vi "Initialize.vi"   [LabVIEW 2011]
uses:
  Controls/Device Cluster.ctl
  GlobalVariables.vi
types:
  T1 = typedef "GP275 Cluster.ctl" = cluster{"Pressure (Torr)":sgl}
  T2 = typedef "RTPC Cluster.ctl" = cluster{"ID Number":u8, "Status":bool[], "Flow (SCCM)":dbl, "Pressure (SCCM)":dbl, "Valve":i16, "Active Instance":i8, "Output":dbl}
  T3 = typedef "MFC Cluster.ctl" = cluster{"ID Number":u8, "Status":bool[], "Flow (SCCM)":dbl, "SetPoint (SCCM)":dbl, "Actuator Override":i8, "Actuator Drive Valve":i16, "Setpoint Output":dbl}
  T4 = typedef "BAR Cluster.ctl" = cluster{"Pressure":dbl}
  T5 = typedef "PC Cluster.ctl" = cluster{"ID Number":u8, "Status":bool[], "Flow (SCCM)":dbl, "SetPoint (SCCM)":dbl, "Actuator Override":i8, "Actuator Drive Valve":i16, "Setpoint Output":dbl}
  T6 = typedef "Device Cluster.ctl" = cluster{"Dnet":string, "Node":i32, "Type":string, "ID Number":u8, "SCCM":dbl, "FullScale":dbl, "Input Bytes":i32, "Output Bytes":i32, "Input Start Location":i32, "Output Start Location":i32, "Enabled":bool, "Bytes":u8[]}
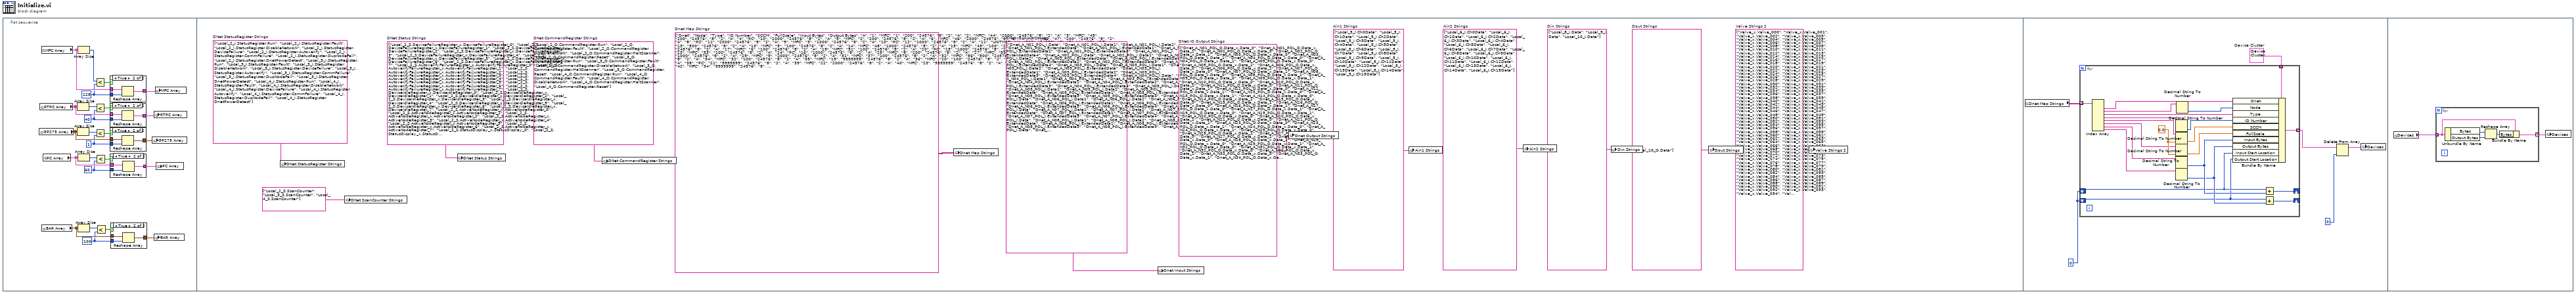
[diagram p0: block diagram]
diagram:
  n1 = flat-sequence {
    frame #0 {
      w2 = 60 ("y")
      w10 = 100 ("y")
      w14 = 1 ("y")
      w18 = 40 ("y")
      w22 = 128 ("y")
      n2 = global read "GlobalVariables.vi" "GP275 Array"() -> (w15:T1[])
      n3 = global read "GlobalVariables.vi" "RTPC Array"() -> (w19:T2[])
      n4 = global read "GlobalVariables.vi" "MFC Array"() -> (w23:T3[])
      n5 = global read "GlobalVariables.vi" "BAR Array"() -> (w11:T4[])
      n6 = global read "GlobalVariables.vi" "PC Array"() -> (w3:T5[])
      n7 = Array Size(array=w19) -> (size(s)=w21:i32)
      n8 = Array Size(array=w15) -> (size(s)=w17:i32)
      n9 = Array Size(array=w3) -> (size(s)=w5:i32)
      n10 = Array Size(array=w23) -> (size(s)=w25:i32)
      n11 = Array Size(array=w11) -> (size(s)=w13:i32)
      n12 = Less?(x=w25, y=w22) -> (x < y?=w24:bool)
      n13 = Less?(x=w21, y=w18) -> (x < y?=w20:bool)
      n14 = Less?(x=w17, y=w14) -> (x < y?=w16:bool)
      n15 = Less?(x=w5, y=w2) -> (x < y?=w4:bool)
      n16 = Less?(x=w13, y=w10) -> (x < y?=w12:bool)
      n17 = case shown="True" w24 {
        tunnel: w23 -> [w42 w45]
        tunnel: w22 -> [_ w44]
        tunnel: [w42 w43] -> w9
        frame False {
        }
        frame True {
          n18 = Reshape Array(w45, w44) -> (w43:T3[])
        }
      }
      n19 = case shown="True" w20 {
        tunnel: w19 -> [w38 w41]
        tunnel: w18 -> [_ w40]
        tunnel: [w38 w39] -> w8
        frame False {
        }
        frame True {
          n20 = Reshape Array(w41, w40) -> (w39:T2[])
        }
      }
      n21 = case shown="True" w16 {
        tunnel: w15 -> [w34 w37]
        tunnel: w14 -> [_ w36]
        tunnel: [w34 w35] -> w7
        frame False {
        }
        frame True {
          n22 = Reshape Array(w37, w36) -> (w35:T1[])
        }
      }
      n23 = case shown="True" w4 {
        tunnel: w3 -> [w26 w29]
        tunnel: w2 -> [_ w28]
        tunnel: [w26 w27] -> w1
        frame False {
        }
        frame True {
          n24 = Reshape Array(w29, w28) -> (w27:T5[])
        }
      }
      n25 = case shown="True" w12 {
        tunnel: w11 -> [w30 w33]
        tunnel: w10 -> [_ w32]
        tunnel: [w30 w31] -> w6
        frame False {
        }
        frame True {
          n26 = Reshape Array(w33, w32) -> (w31:T4[])
        }
      }
      n27 = global write "GlobalVariables.vi" "GP275 Array"(w7) -> ()
      n28 = global write "GlobalVariables.vi" "RTPC Array"(w8) -> ()
      n29 = global write "GlobalVariables.vi" "BAR Array"(w6) -> ()
      n30 = global write "GlobalVariables.vi" "MFC Array"(w9) -> ()
      n31 = global write "GlobalVariables.vi" "PC Array"(w1) -> ()
    }
    frame #1 {
      w47 = string[] ["Dnet_A_N01_POL_O.Data_x.Data_0", "Dnet_A_N01_POL_O.Data_x.Data_1", "Dnet_A_N02_POL_O.Data_x.Data_0", "Dnet_A_N02_POL_O.Data_x.Data_1", "Dnet_A_N03_POL_O.Data_x.Data_0", "Dnet_A_N03_POL_O.Data_x.Data_1", "Dnet_A_N04_POL_O.Data_x.Data_0", "Dnet_A_N04_POL_O.Data_x.Data_1", "Dnet_A_N05_POL_O.Data_x.Data_0", "Dnet_A_N05_POL_O.Data_x.Data_1", "Dnet_A_N06_POL_O.Data_x.Data_0", "Dnet_A_N06_POL_O.Data_x.Data_1", "Dnet_A_N07_POL_O.Data_x.Data_0", "Dnet_A_N07_POL_O.Data_x.Data_1", "Dnet_A_N08_POL_O.Data_x.Data_0", "Dnet_A_N08_POL_O.Data_x.Data_1", "Dnet_A_N09_POL_O.Data_x.Data_0", "Dnet_A_N09_POL_O.Data_x.Data_1", "Dnet_A_N10_POL_O.Data_x.Data_0", "Dnet_A_N10_POL_O.Data_x.Data_1", "Dnet_A_N11_POL_O.Data_x.Data_0", "Dnet_A_N11_POL_O.Data_x.Data_1", "Dnet_A_N12_POL_O.Data_x.Data_0", "Dnet_A_N12_POL_O.Data_x.Data_1", "Dnet_A_N13_POL_O.Data_x.Data_0", "Dnet_A_N13_POL_O.Data_x.Data_1", "Dnet_A_N14_POL_O.Data_x.Data_0", "Dnet_A_N14_POL_O.Data_x.Data_1", "Dnet_A_N15_POL_O.Data_x.Data_0", "Dnet_A_N15_POL_O.Data_x.Data_1", "Dnet_A_N16_POL_O.Data_x.Data_0", "Dnet_A_N16_POL_O.Data_x.Data_1", "Dnet_A_N17_POL_O.Data_x.Data_0", "Dnet_A_N17_POL_O.Data_x.Data_1", "Dnet_A_N19_POL_O.Data_x.Data_0", "Dnet_A_N19_POL_O.Data_x.Data_1", "Dnet_A_N20_POL_O.Data_x.Data_0", "Dnet_A_N20_POL_O.Data_x.Data_1", "Dnet_A_N21_POL_O.Data_x.Data_0", "Dnet_A_N21_POL_O.Data_x.Data_1", "Dnet_A_N23_POL_O.Data_x.Data_0", "Dnet_A_N23_POL_O.Data_x.Data_1", "Dnet_A_N24_POL_O.Data_x.Data_0", "Dnet_A_N24_POL_O.Data_x.Data_1", "Dnet_A_N25_POL_O.Data_x.Data_0", "Dnet_A_N25_POL_O.Data_x.Data_1", "Dnet_A_N27_POL_O.Data_x.Data_0", "Dnet_A_N27_POL_O.Data_x.Data_1", "Dnet_A_N28_POL_O.Data_x.Data_0", "Dnet_A_N28_POL_O.Data_x.Data_1", "Dnet_A_N29_POL_O.Data_x.Data_0", "Dnet_A_N29_POL_O.Data_x.Data_1", "Dnet_A_N31_POL_O.Data_x.Data_0", "Dnet_A_N31_POL_O.Data_x.Data_1", "Dnet_A_N32_POL_O.Data_x.Data_0", "Dnet_A_N32_POL_O.Data_x.Data_1", "Dnet_A_N33_POL_O.Data_x.Data_0", "Dnet_A_N33_POL_O.Data_x.Data_1", "Dnet_A_N34_POL_O.Data_x.Data_0", "Dnet_A_N34_POL_O.Data_x.Data_1", "Dnet_A_N35_POL_O.Data_x.Data_0", "Dnet_A_N35_POL_O.Data_x.Data_1", "Dnet_A_N36_POL_O.Data_x.Data_0", "Dnet_A_N36_POL_O.Data_x.Data_1", "Dnet_A_N37_POL_O.Data_x.Data_0", "Dnet_A_N37_POL_O.Data_x.Data_1", "Dnet_A_N38_POL_O.Data_x.Data_0", "Dnet_A_N38_POL_O.Data_x.Data_1", "Dnet_A_N39_POL_O.Data_x.Data_0", "Dnet_A_N39_POL_O.Data_x.Data_1", "Dnet_A_N40_POL_O.Data_x.Data_0", "Dnet_A_N40_POL_O.Data_x.Data_1", "Dnet_A_N41_POL_O.Data_x.Data_0", "Dnet_A_N41_POL_O.Data_x.Data_1", "Dnet_A_N42_POL_O.Data_x.Data_0", "Dnet_A_N42_POL_O.Data_x.Data_1", "Dnet_A_N43_POL_O.Data_x.Data_0", "Dnet_A_N43_POL_O.Data_x.Data_1", "Dnet_A_N44_POL_O.Data_x.Data_0", "Dnet_A_N44_POL_O.Data_x.Data_1", "Dnet_A_N45_POL_O.Data_x.Data_0", "Dnet_A_N45_POL_O.Data_x.Data_1", "Dnet_A_N46_POL_O.Data_x.Data_0", "Dnet_A_N46_POL_O.Data_x.Data_1", "Dnet_A_N47_POL_O.Data_x.Data_0", "Dnet_A_N47_POL_O.Data_x.Data_1", "Dnet_A_N49_POL_O.Data", "Dnet_A_N49_POL_O.Data1", "Dnet_A_N49_POL_O.ExtendedData", "Dnet_A_N50_POL_O.Data_x.Data_0", "Dnet_A_N50_POL_O.Data_x.Data_1", "Dnet_A_N51_POL_O.Data_x.Data_0", "Dnet_A_N51_POL_O.Data_x.Data_1", "Dnet_A_N52_POL_O.Data", "Dnet_A_N52_POL_O.Data1", "Dnet_A_N52_POL_O.ExtendedData", "Dnet_A_N53_POL_O.Data", "Dnet_A_N53_POL_O.Data1", "Dnet_A_N53_POL_O.ExtendedData", "Dnet_A_N54_POL_O.Data", "Dnet_A_N54_POL_O.Data1", "Dnet_A_N54_POL_O.ExtendedData", "Dnet_A_N55_POL_O.Data_x.Data_0", "Dnet_A_N55_POL_O.Data_x.Data_1", "Dnet_A_N56_POL_O.Data_x.Data_0", "Dnet_A_N56_POL_O.Data_x.Data_1", "Dnet_A_N60_POL_O.Data_x.Data_0", "Dnet_A_N60_POL_O.Data_x.Data_1", "Dnet_A_N60_POL_O.Data_x.Data_2", "Dnet_A_N60_POL_O.Data_x.Data_3", "Dnet_A_N60_POL_O.Data_x.Data_4", "Dnet_A_N60_POL_O.Data_x.Data_5", "Dnet_A_N60_POL_O.Data_x.Data_6", "Dnet_A_N60_POL_O.Data_x.Data_7", "Dnet_A_N63_POL_O.Data_x.Data_0", "Dnet_A_N63_POL_O.Data_x.Data_1", "Dnet_B_N01_POL_O.Data_x.Data_0", "Dnet_B_N01_POL_O.Data_x.Data_1", "Dnet_B_N02_POL_O.Data_x.Data_0", "Dnet_B_N02_POL_O.Data_x.Data_1", "Dnet_B_N03_POL_O.Data_x.Data_0", "Dnet_B_N03_POL_O.Data_x.Data_1", "Dnet_B_N04_POL_O.Data_x.Data_0", "Dnet_B_N04_POL_O.Data_x.Data_1", "Dnet_B_N05_POL_O.Data_x.Data_0", "Dnet_B_N05_POL_O.Data_x.Data_1", "Dnet_B_N06_POL_O.Data_x.Data_0", "Dnet_B_N06_POL_O.Data_x.Data_1", "Dnet_B_N08_POL_O.Data_x.Data_0", "Dnet_B_N08_POL_O.Data_x.Data_1", "Dnet_B_N09_POL_O.Data_x.Data_0", "Dnet_B_N09_POL_O.Data_x.Data_1", "Dnet_B_N10_POL_O.Data_x.Data_0", "Dnet_B_N10_POL_O.Data_x.Data_1", "Dnet_B_N11_POL_O.Data_x.Data_0", "Dnet_B_N11_POL_O.Data_x.Data_1", "Dnet_B_N12_POL_O.Data_x.Data_0", "Dnet_B_N12_POL_O.Data_x.Data_1", "Dnet_B_N13_POL_O.Data_x.Data_0", "Dnet_B_N13_POL_O.Data_x.Data_1", "Dnet_B_N14_POL_O.Data_x.Data_0", "Dnet_B_N14_POL_O.Data_x.Data_1", "Dnet_B_N15_POL_O.Data_x.Data_0", "Dnet_B_N15_POL_O.Data_x.Data_1", "Dnet_B_N21_POL_O.Data", "Dnet_C_N09_POL_O.Data_x.Data_00", "Dnet_C_N09_POL_O.Data_x.Data_01", "Dnet_C_N09_POL_O.Data_x.Data_02", "Dnet_C_N09_POL_O.Data_x.Data_03", "Dnet_C_N09_POL_O.Data_x.Data_04", "Dnet_C_N09_POL_O.Data_x.Data_05", "Dnet_C_N09_POL_O.Data_x.Data_06", "Dnet_C_N09_POL_O.Data_x.Data_07", "Dnet_C_N09_POL_O.Data_x.Data_08", "Dnet_C_N09_POL_O.Data_x.Data_09", "Dnet_C_N09_POL_O.Data_x.Data_10", "Dnet_C_N09_POL_O.Data_x.Data_11", "Dnet_C_N09_POL_O.Data_x.Data_12", "Dnet_C_N09_POL_O.Data_x.Data_13", "Dnet_C_N09_POL_O.Data_x.Data_14", "Dnet_C_N09_POL_O.Data_x.Data_15", "Dnet_C_N09_POL_O.Data_x.Data_16", "Dnet_C_N09_POL_O.Data_x.Data_17", "Dnet_C_N09_POL_O.Data_x.Data_18", "Dnet_C_N09_POL_O.Data_x.Data_19", "Dnet_C_N09_POL_O.Data_x.Data_20", "Dnet_C_N09_POL_O.Data_x.Data_21", "Dnet_C_N09_POL_O.Data_x.Data_22", "Dnet_C_N09_POL_O.Data_x.Data_23", "Dnet_C_N09_POL_O.Data_x.Data_24", "Dnet_C_N09_POL_O.Data_x.Data_25", "Dnet_C_N09_POL_O.Data_x.Data_26", "Dnet_C_N09_POL_O.Data_x.Data_27", "Dnet_C_N09_POL_O.Data_x.Data_28", "Dnet_C_N09_POL_O.Data_x.Data_29", "Dnet_C_N09_POL_O.Data_x.Data_30", "Dnet_C_N09_POL_O.Data_x.Data_31", "Dnet_C_N09_POL_O.Data_x.Data_32", "Dnet_C_N09_POL_O.Data_x.Data_33", "Dnet_C_N09_POL_O.Data_x.Data_34", "Dnet_C_N09_POL_O.Data_x.Data_35", "Dnet_C_N09_POL_O.Data_x.Data_36", "Dnet_C_N09_POL_O.Data_x.Data_37", "Dnet_C_N09_POL_O.Data_x.Data_38", "Dnet_C_N09_POL_O.Data_x.Data_39", "Dnet_C_N09_POL_O.Data_x.Data_40", "Dnet_C_N09_POL_O.Data_x.Data_41", "Dnet_C_N09_POL_O.Data_x.Data_42", "Dnet_C_N09_POL_O.Data_x.Data_43", "Dnet_C_N09_POL_O.Data_x.Data_44", "Dnet_C_N09_POL_O.Data_x.Data_45", "Dnet_C_N09_POL_O.Data_x.Data_46", "Dnet_C_N09_POL_O.Data_x.Data_47", "Dnet_C_N09_POL_O.Data_x.Data_48", "Dnet_C_N09_POL_O.Data_x.Data_49", "Dnet_C_N09_POL_O.Data_x.Data_50", "Dnet_C_N09_POL_O.Data_x.Data_51", "Dnet_C_N09_POL_O.Data_x.Data_52", "Dnet_C_N09_POL_O.Data_x.Data_53", "Dnet_C_N09_POL_O.Data_x.Data_54", "Dnet_C_N09_POL_O.Data_x.Data_55", "Dnet_C_N09_POL_O.Data_x.Data_56", "Dnet_C_N09_POL_O.Data_x.Data_57", "Dnet_C_N09_POL_O.Data_x.Data_58", "Dnet_C_N09_POL_O.Data_x.Data_59", "Dnet_C_N09_POL_O.Data_x.Data_60", "Dnet_C_N09_POL_O.Data_x.Data_61", "Dnet_C_N09_POL_O.Data_x.Data_62", "Dnet_C_N09_POL_O.Data_x.Data_63", "Dnet_C_N09_POL_O.Data_x.Data_64", "Dnet_C_N09_POL_O.Data_x.Data_65", "Dnet_C_N09_POL_O.Data_x.Data_66", "Dnet_C_N09_POL_O.Data_x.Data_67", "Dnet_C_N09_POL_O.Data_x.Data_68", "Dnet_C_N09_POL_O.Data_x.Data_69", "Dnet_C_N09_POL_O.Data_x.Data_70", "Dnet_C_N09_POL_O.Data_x.Data_71", "Dnet_C_N09_POL_O.Data_x.Data_72", "Dnet_C_N09_POL_O.Data_x.Data_73", "Dnet_C_N09_POL_O.Data_x.Data_74", "Dnet_C_N09_POL_O.Data_x.Data_75", "Dnet_C_N09_POL_O.Data_x.Data_76", "Dnet_C_N09_POL_O.Data_x.Data_77", "Dnet_C_N09_POL_O.Data_x.Data_78", "Dnet_C_N09_POL_O.Data_x.Data_79"]  # DNet IO Output Strings
      w46 = string[] ["Dnet_A_N01_POL_I.Data", "Dnet_A_N01_POL_I.Data1", "Dnet_A_N01_POL_I.Data2", "Dnet_A_N01_POL_I.ExtendedData", "Dnet_A_N01_POL_I.ExtendedData1", "Dnet_A_N01_POL_I.ExtendedData2", "Dnet_A_N01_POL_I.ExtendedData3", "Dnet_A_N01_POL_I.ExtendedData4", "Dnet_A_N02_POL_I.Data", "Dnet_A_N02_POL_I.Data1", "Dnet_A_N02_POL_I.Data2", "Dnet_A_N02_POL_I.ExtendedData", "Dnet_A_N02_POL_I.ExtendedData1", "Dnet_A_N02_POL_I.ExtendedData2", "Dnet_A_N02_POL_I.ExtendedData3", "Dnet_A_N02_POL_I.ExtendedData4", "Dnet_A_N03_POL_I.Data", "Dnet_A_N03_POL_I.Data1", "Dnet_A_N03_POL_I.Data2", "Dnet_A_N03_POL_I.ExtendedData", "Dnet_A_N03_POL_I.ExtendedData1", "Dnet_A_N03_POL_I.ExtendedData2", "Dnet_A_N03_POL_I.ExtendedData3", "Dnet_A_N03_POL_I.ExtendedData4", "Dnet_A_N04_POL_I.Data", "Dnet_A_N04_POL_I.Data1", "Dnet_A_N04_POL_I.Data2", "Dnet_A_N04_POL_I.ExtendedData", "Dnet_A_N04_POL_I.ExtendedData1", "Dnet_A_N04_POL_I.ExtendedData2", "Dnet_A_N04_POL_I.ExtendedData3", "Dnet_A_N04_POL_I.ExtendedData4", "Dnet_A_N05_POL_I.Data", "Dnet_A_N05_POL_I.Data1", "Dnet_A_N05_POL_I.Data2", "Dnet_A_N05_POL_I.ExtendedData", "Dnet_A_N05_POL_I.ExtendedData1", "Dnet_A_N05_POL_I.ExtendedData2", "Dnet_A_N05_POL_I.ExtendedData3", "Dnet_A_N05_POL_I.ExtendedData4", "Dnet_A_N06_POL_I.Data", "Dnet_A_N06_POL_I.Data1", "Dnet_A_N06_POL_I.Data2", "Dnet_A_N06_POL_I.ExtendedData", "Dnet_A_N06_POL_I.ExtendedData1", "Dnet_A_N06_POL_I.ExtendedData2", "Dnet_A_N06_POL_I.ExtendedData3", "Dnet_A_N06_POL_I.ExtendedData4", "Dnet_A_N07_POL_I.Data", "Dnet_A_N07_POL_I.Data1", "Dnet_A_N07_POL_I.Data2", "Dnet_A_N07_POL_I.ExtendedData", "Dnet_A_N07_POL_I.ExtendedData1", "Dnet_A_N07_POL_I.ExtendedData2", "Dnet_A_N07_POL_I.ExtendedData3", "Dnet_A_N07_POL_I.ExtendedData4", "Dnet_A_N08_POL_I.Data", "Dnet_A_N08_POL_I.Data1", "Dnet_A_N08_POL_I.Data2", "Dnet_A_N08_POL_I.ExtendedData", "Dnet_A_N08_POL_I.ExtendedData1", "Dnet_A_N08_POL_I.ExtendedData2", "Dnet_A_N08_POL_I.ExtendedData3", "Dnet_A_N08_POL_I.ExtendedData4", "Dnet_A_N09_POL_I.Data", "Dnet_A_N09_POL_I.Data1", "Dnet_A_N09_POL_I.Data2", "Dnet_A_N09_POL_I.ExtendedData", "Dnet_A_N09_POL_I.ExtendedData1", "Dnet_A_N09_POL_I.ExtendedData2", "Dnet_A_N09_POL_I.ExtendedData3", "Dnet_A_N09_POL_I.ExtendedData4", "Dnet_A_N10_POL_I.Data", "Dnet_A_N10_POL_I.Data1", "Dnet_A_N10_POL_I.Data2", "Dnet_A_N10_POL_I.ExtendedData", "Dnet_A_N10_POL_I.ExtendedData1", "Dnet_A_N10_POL_I.ExtendedData2", "Dnet_A_N10_POL_I.ExtendedData3", "Dnet_A_N10_POL_I.ExtendedData4", "Dnet_A_N11_POL_I.Data_x.Data_0", "Dnet_A_N11_POL_I.Data_x.Data_1", "Dnet_A_N11_POL_I.Data_x.Data_2", "Dnet_A_N11_POL_I.Data_x.Data_3", "Dnet_A_N11_POL_I.Data_x.Data_4", "Dnet_A_N11_POL_I.Data_x.Data_5", "Dnet_A_N11_POL_I.Data_x.Data_6", "Dnet_A_N11_POL_I.Data_x.Data_7", "Dnet_A_N12_POL_I.Data", "Dnet_A_N12_POL_I.Data1", "Dnet_A_N12_POL_I.Data2", "Dnet_A_N12_POL_I.ExtendedData", "Dnet_A_N12_POL_I.ExtendedData1", "Dnet_A_N12_POL_I.ExtendedData2", "Dnet_A_N12_POL_I.ExtendedData3", "Dnet_A_N12_POL_I.ExtendedData4", "Dnet_A_N13_POL_I.Data", "Dnet_A_N13_POL_I.Data1", "Dnet_A_N13_POL_I.Data2", "Dnet_A_N13_POL_I.ExtendedData", "Dnet_A_N13_POL_I.ExtendedData1", "Dnet_A_N13_POL_I.ExtendedData2", "Dnet_A_N13_POL_I.ExtendedData3", "Dnet_A_N13_POL_I.ExtendedData4", "Dnet_A_N14_POL_I.Data", "Dnet_A_N14_POL_I.Data1", "Dnet_A_N14_POL_I.Data2", "Dnet_A_N14_POL_I.ExtendedData", "Dnet_A_N14_POL_I.ExtendedData1", "Dnet_A_N14_POL_I.ExtendedData2", "Dnet_A_N14_POL_I.ExtendedData3", "Dnet_A_N14_POL_I.ExtendedData4", "Dnet_A_N15_POL_I.Data", "Dnet_A_N15_POL_I.Data1", "Dnet_A_N15_POL_I.Data2", "Dnet_A_N15_POL_I.ExtendedData", "Dnet_A_N15_POL_I.ExtendedData1", "Dnet_A_N15_POL_I.ExtendedData2", "Dnet_A_N15_POL_I.ExtendedData3", "Dnet_A_N15_POL_I.ExtendedData4", "Dnet_A_N16_POL_I.Data", "Dnet_A_N16_POL_I.Data1", "Dnet_A_N16_POL_I.Data2", "Dnet_A_N16_POL_I.ExtendedData", "Dnet_A_N16_POL_I.ExtendedData1", "Dnet_A_N16_POL_I.ExtendedData2", "Dnet_A_N16_POL_I.ExtendedData3", "Dnet_A_N16_POL_I.ExtendedData4", "Dnet_A_N17_POL_I.Data", "Dnet_A_N17_POL_I.Data1", "Dnet_A_N17_POL_I.Data2", "Dnet_A_N17_POL_I.ExtendedData", "Dnet_A_N17_POL_I.ExtendedData1", "Dnet_A_N17_POL_I.ExtendedData2", "Dnet_A_N17_POL_I.ExtendedData3", "Dnet_A_N17_POL_I.ExtendedData4", "Dnet_A_N19_POL_I.Data", "Dnet_A_N19_POL_I.Data1", "Dnet_A_N19_POL_I.Data2", "Dnet_A_N19_POL_I.ExtendedData", "Dnet_A_N19_POL_I.ExtendedData1", "Dnet_A_N19_POL_I.ExtendedData2", "Dnet_A_N19_POL_I.ExtendedData3", "Dnet_A_N19_POL_I.ExtendedData4", "Dnet_A_N20_POL_I.Data", "Dnet_A_N20_POL_I.Data1", "Dnet_A_N20_POL_I.Data2", "Dnet_A_N20_POL_I.ExtendedData", "Dnet_A_N20_POL_I.ExtendedData1", "Dnet_A_N20_POL_I.ExtendedData2", "Dnet_A_N20_POL_I.ExtendedData3", "Dnet_A_N20_POL_I.ExtendedData4", "Dnet_A_N21_POL_I.Data", "Dnet_A_N21_POL_I.Data1", "Dnet_A_N21_POL_I.Data2", "Dnet_A_N21_POL_I.ExtendedData", "Dnet_A_N21_POL_I.ExtendedData1", "Dnet_A_N21_POL_I.ExtendedData2", "Dnet_A_N21_POL_I.ExtendedData3", "Dnet_A_N21_POL_I.ExtendedData4", "Dnet_A_N23_POL_I.Data", "Dnet_A_N23_POL_I.Data1", "Dnet_A_N23_POL_I.Data2", "Dnet_A_N23_POL_I.ExtendedData", "Dnet_A_N23_POL_I.ExtendedData1", "Dnet_A_N23_POL_I.ExtendedData2", "Dnet_A_N23_POL_I.ExtendedData3", "Dnet_A_N23_POL_I.ExtendedData4", "Dnet_A_N24_POL_I.Data", "Dnet_A_N24_POL_I.Data1", "Dnet_A_N24_POL_I.Data2", "Dnet_A_N24_POL_I.ExtendedData", "Dnet_A_N24_POL_I.ExtendedData1", "Dnet_A_N24_POL_I.ExtendedData2", "Dnet_A_N24_POL_I.ExtendedData3", "Dnet_A_N24_POL_I.ExtendedData4", "Dnet_A_N25_POL_I.Data", "Dnet_A_N25_POL_I.Data1", "Dnet_A_N25_POL_I.Data2", "Dnet_A_N25_POL_I.ExtendedData", "Dnet_A_N25_POL_I.ExtendedData1", "Dnet_A_N25_POL_I.ExtendedData2", "Dnet_A_N25_POL_I.ExtendedData3", "Dnet_A_N25_POL_I.ExtendedData4", "Dnet_A_N27_POL_I.Data", "Dnet_A_N27_POL_I.Data1", "Dnet_A_N27_POL_I.Data2", "Dnet_A_N27_POL_I.ExtendedData", "Dnet_A_N27_POL_I.ExtendedData1", "Dnet_A_N27_POL_I.ExtendedData2", "Dnet_A_N27_POL_I.ExtendedData3", "Dnet_A_N27_POL_I.ExtendedData4", "Dnet_A_N28_POL_I.Data", "Dnet_A_N28_POL_I.Data1", "Dnet_A_N28_POL_I.Data2", "Dnet_A_N28_POL_I.ExtendedData", "Dnet_A_N28_POL_I.ExtendedData1", "Dnet_A_N28_POL_I.ExtendedData2", "Dnet_A_N28_POL_I.ExtendedData3", "Dnet_A_N28_POL_I.ExtendedData4", "Dnet_A_N29_POL_I.Data", "Dnet_A_N29_POL_I.Data1", "Dnet_A_N29_POL_I.Data2", "Dnet_A_N29_POL_I.ExtendedData", "Dnet_A_N29_POL_I.ExtendedData1", "Dnet_A_N29_POL_I.ExtendedData2", "Dnet_A_N29_POL_I.ExtendedData3", "Dnet_A_N29_POL_I.ExtendedData4", "Dnet_A_N31_POL_I.Data", "Dnet_A_N31_POL_I.Data1", "Dnet_A_N31_POL_I.Data2", "Dnet_A_N31_POL_I.ExtendedData", "Dnet_A_N31_POL_I.ExtendedData1", "Dnet_A_N31_POL_I.ExtendedData2", "Dnet_A_N31_POL_I.ExtendedData3", "Dnet_A_N31_POL_I.ExtendedData4", "Dnet_A_N32_POL_I.Data", "Dnet_A_N32_POL_I.Data1", "Dnet_A_N32_POL_I.Data2", "Dnet_A_N32_POL_I.ExtendedData", "Dnet_A_N32_POL_I.ExtendedData1", "Dnet_A_N32_POL_I.ExtendedData2", "Dnet_A_N32_POL_I.ExtendedData3", "Dnet_A_N32_POL_I.ExtendedData4", "Dnet_A_N33_POL_I.Data", "Dnet_A_N33_POL_I.Data1", "Dnet_A_N33_POL_I.Data2", "Dnet_A_N33_POL_I.ExtendedData", "Dnet_A_N33_POL_I.ExtendedData1", "Dnet_A_N33_POL_I.ExtendedData2", "Dnet_A_N33_POL_I.ExtendedData3", "Dnet_A_N33_POL_I.ExtendedData4", "Dnet_A_N34_POL_I.Data", "Dnet_A_N34_POL_I.Data1", "Dnet_A_N34_POL_I.Data2", "Dnet_A_N34_POL_I.ExtendedData", "Dnet_A_N34_POL_I.ExtendedData1", "Dnet_A_N34_POL_I.ExtendedData2", "Dnet_A_N34_POL_I.ExtendedData3", "Dnet_A_N34_POL_I.ExtendedData4", "Dnet_A_N35_POL_I.Data", "Dnet_A_N35_POL_I.Data1", "Dnet_A_N35_POL_I.Data2", "Dnet_A_N35_POL_I.ExtendedData", "Dnet_A_N35_POL_I.ExtendedData1", "Dnet_A_N35_POL_I.ExtendedData2", "Dnet_A_N35_POL_I.ExtendedData3", "Dnet_A_N35_POL_I.ExtendedData4", "Dnet_A_N36_POL_I.Data", "Dnet_A_N36_POL_I.Data1", "Dnet_A_N36_POL_I.Data2", "Dnet_A_N36_POL_I.ExtendedData", "Dnet_A_N36_POL_I.ExtendedData1", "Dnet_A_N36_POL_I.ExtendedData2", "Dnet_A_N36_POL_I.ExtendedData3", "Dnet_A_N36_POL_I.ExtendedData4", "Dnet_A_N37_POL_I.Data_x.Data_0", "Dnet_A_N37_POL_I.Data_x.Data_1", "Dnet_A_N37_POL_I.Data_x.Data_2", "Dnet_A_N37_POL_I.Data_x.Data_3", "Dnet_A_N37_POL_I.Data_x.Data_4", "Dnet_A_N37_POL_I.Data_x.Data_5", "Dnet_A_N37_POL_I.Data_x.Data_6", "Dnet_A_N37_POL_I.Data_x.Data_7", "Dnet_A_N38_POL_I.Data", "Dnet_A_N38_POL_I.Data1", "Dnet_A_N38_POL_I.Data2", "Dnet_A_N38_POL_I.ExtendedData", "Dnet_A_N38_POL_I.ExtendedData1", "Dnet_A_N38_POL_I.ExtendedData2", "Dnet_A_N38_POL_I.ExtendedData3", "Dnet_A_N38_POL_I.ExtendedData4", "Dnet_A_N39_POL_I.Data", "Dnet_A_N39_POL_I.Data1", "Dnet_A_N39_POL_I.Data2", "Dnet_A_N39_POL_I.ExtendedData", "Dnet_A_N39_POL_I.ExtendedData1", "Dnet_A_N39_POL_I.ExtendedData2", "Dnet_A_N39_POL_I.ExtendedData3", "Dnet_A_N39_POL_I.ExtendedData4", "Dnet_A_N40_POL_I.Data", "Dnet_A_N40_POL_I.Data1", "Dnet_A_N40_POL_I.Data2", "Dnet_A_N40_POL_I.ExtendedData", "Dnet_A_N40_POL_I.ExtendedData1", "Dnet_A_N40_POL_I.ExtendedData2", "Dnet_A_N40_POL_I.ExtendedData3", "Dnet_A_N40_POL_I.ExtendedData4", "Dnet_A_N41_POL_I.Data", "Dnet_A_N41_POL_I.Data1", "Dnet_A_N41_POL_I.Data2", "Dnet_A_N41_POL_I.ExtendedData", "Dnet_A_N41_POL_I.ExtendedData1", "Dnet_A_N41_POL_I.ExtendedData2", "Dnet_A_N41_POL_I.ExtendedData3", "Dnet_A_N41_POL_I.ExtendedData4", "Dnet_A_N42_POL_I.Data", "Dnet_A_N42_POL_I.Data1", "Dnet_A_N42_POL_I.Data2", "Dnet_A_N42_POL_I.ExtendedData", "Dnet_A_N42_POL_I.ExtendedData1", "Dnet_A_N42_POL_I.ExtendedData2", "Dnet_A_N42_POL_I.ExtendedData3", "Dnet_A_N42_POL_I.ExtendedData4", "Dnet_A_N43_POL_I.Data", "Dnet_A_N43_POL_I.Data1", "Dnet_A_N43_POL_I.Data2", "Dnet_A_N43_POL_I.ExtendedData", "Dnet_A_N43_POL_I.ExtendedData1", "Dnet_A_N43_POL_I.ExtendedData2", "Dnet_A_N43_POL_I.ExtendedData3", "Dnet_A_N43_POL_I.ExtendedData4", "Dnet_A_N44_POL_I.Data", "Dnet_A_N44_POL_I.Data1", "Dnet_A_N44_POL_I.Data2", "Dnet_A_N44_POL_I.ExtendedData", "Dnet_A_N44_POL_I.ExtendedData1", "Dnet_A_N44_POL_I.ExtendedData2", "Dnet_A_N44_POL_I.ExtendedData3", "Dnet_A_N44_POL_I.ExtendedData4", "Dnet_A_N45_POL_I.Data", "Dnet_A_N45_POL_I.Data1", "Dnet_A_N45_POL_I.Data2", "Dnet_A_N45_POL_I.ExtendedData", "Dnet_A_N45_POL_I.ExtendedData1", "Dnet_A_N45_POL_I.ExtendedData2", "Dnet_A_N45_POL_I.ExtendedData3", "Dnet_A_N45_POL_I.ExtendedData4", "Dnet_A_N46_POL_I.Data", "Dnet_A_N46_POL_I.Data1", "Dnet_A_N46_POL_I.Data2", "Dnet_A_N46_POL_I.ExtendedData", "Dnet_A_N46_POL_I.ExtendedData1", "Dnet_A_N46_POL_I.ExtendedData2", "Dnet_A_N46_POL_I.ExtendedData3", "Dnet_A_N46_POL_I.ExtendedData4", "Dnet_A_N47_POL_I.Data", "Dnet_A_N47_POL_I.Data1", "Dnet_A_N47_POL_I.Data2", "Dnet_A_N47_POL_I.ExtendedData", "Dnet_A_N47_POL_I.ExtendedData1", "Dnet_A_N47_POL_I.ExtendedData2", "Dnet_A_N47_POL_I.ExtendedData3", "Dnet_A_N47_POL_I.ExtendedData4", "Dnet_A_N48_POL_I.Data_x.Data_0", "Dnet_A_N48_POL_I.Data_x.Data_1", "Dnet_A_N48_POL_I.Data_x.Data_2", "Dnet_A_N49_POL_I.Data", "Dnet_A_N49_POL_I.Data1", "Dnet_A_N49_POL_I.Data2", "Dnet_A_N49_POL_I.ExtendedData", "Dnet_A_N49_POL_I.ExtendedData1", "Dnet_A_N49_POL_I.ExtendedData2", "Dnet_A_N49_POL_I.ExtendedData3", "Dnet_A_N49_POL_I.ExtendedData4", "Dnet_A_N50_POL_I.Data_x.Data_0", "Dnet_A_N50_POL_I.Data_x.Data_1", "Dnet_A_N50_POL_I.Data_x.Data_2", "Dnet_A_N50_POL_I.Data_x.Data_3", "Dnet_A_N50_POL_I.Data_x.Data_4", "Dnet_A_N50_POL_I.Data_x.Data_5", "Dnet_A_N50_POL_I.Data_x.Data_6", "Dnet_A_N50_POL_I.Data_x.Data_7", "Dnet_A_N51_POL_I.Data_x.Data_0", "Dnet_A_N51_POL_I.Data_x.Data_1", "Dnet_A_N51_POL_I.Data_x.Data_2", "Dnet_A_N51_POL_I.Data_x.Data_3", "Dnet_A_N51_POL_I.Data_x.Data_4", "Dnet_A_N51_POL_I.Data_x.Data_5", "Dnet_A_N51_POL_I.Data_x.Data_6", "Dnet_A_N51_POL_I.Data_x.Data_7", "Dnet_A_N52_POL_I.Data", "Dnet_A_N52_POL_I.Data1", "Dnet_A_N52_POL_I.Data2", "Dnet_A_N52_POL_I.ExtendedData", "Dnet_A_N52_POL_I.ExtendedData1", "Dnet_A_N52_POL_I.ExtendedData2", "Dnet_A_N52_POL_I.ExtendedData3", "Dnet_A_N52_POL_I.ExtendedData4", "Dnet_A_N53_POL_I.Data", "Dnet_A_N53_POL_I.Data1", "Dnet_A_N53_POL_I.Data2", "Dnet_A_N53_POL_I.ExtendedData", "Dnet_A_N53_POL_I.ExtendedData1", "Dnet_A_N53_POL_I.ExtendedData2", "Dnet_A_N53_POL_I.ExtendedData3", "Dnet_A_N53_POL_I.ExtendedData4", "Dnet_A_N54_POL_I.Data", "Dnet_A_N54_POL_I.Data1", "Dnet_A_N54_POL_I.Data2", "Dnet_A_N54_POL_I.ExtendedData", "Dnet_A_N54_POL_I.ExtendedData1", "Dnet_A_N54_POL_I.ExtendedData2", "Dnet_A_N54_POL_I.ExtendedData3", "Dnet_A_N54_POL_I.ExtendedData4", "Dnet_A_N55_POL_I.Data", "Dnet_A_N55_POL_I.Data1", "Dnet_A_N55_POL_I.Data2", "Dnet_A_N55_POL_I.ExtendedData", "Dnet_A_N55_POL_I.ExtendedData1", "Dnet_A_N55_POL_I.ExtendedData2", "Dnet_A_N55_POL_I.ExtendedData3", "Dnet_A_N55_POL_I.ExtendedData4", "Dnet_A_N56_POL_I.Data", "Dnet_A_N56_POL_I.Data1", "Dnet_A_N56_POL_I.Data2", "Dnet_A_N56_POL_I.ExtendedData", "Dnet_A_N56_POL_I.ExtendedData1", "Dnet_A_N56_POL_I.ExtendedData2", "Dnet_A_N56_POL_I.ExtendedData3", "Dnet_A_N56_POL_I.ExtendedData4", "Dnet_A_N60_POL_I.Data_x.Data_0", "Dnet_A_N60_POL_I.Data_x.Data_1", "Dnet_A_N60_POL_I.Data_x.Data_2", "Dnet_A_N60_POL_I.Data_x.Data_3", "Dnet_A_N60_POL_I.Data_x.Data_4", "Dnet_A_N60_POL_I.Data_x.Data_5", "Dnet_A_N60_POL_I.Data_x.Data_6", "Dnet_A_N60_POL_I.Data_x.Data_7", "Dnet_A_N61_POL_I.Data_x.Data_0", "Dnet_A_N61_POL_I.Data_x.Data_1", "Dnet_A_N61_POL_I.Data_x.Data_2", "Dnet_A_N63_POL_I.Data", "Dnet_A_N63_POL_I.Data1", "Dnet_A_N63_POL_I.Data2", "Dnet_A_N63_POL_I.ExtendedData", "Dnet_A_N63_POL_I.ExtendedData1", "Dnet_A_N63_POL_I.ExtendedData2", "Dnet_A_N63_POL_I.ExtendedData3", "Dnet_A_N63_POL_I.ExtendedData4", "Dnet_B_N01_POL_I.Data", "Dnet_B_N01_POL_I.Data1", "Dnet_B_N01_POL_I.Data2", "Dnet_B_N01_POL_I.ExtendedData", "Dnet_B_N01_POL_I.ExtendedData1", "Dnet_B_N01_POL_I.ExtendedData2", "Dnet_B_N01_POL_I.ExtendedData3", "Dnet_B_N01_POL_I.ExtendedData4", "Dnet_B_N02_POL_I.Data", "Dnet_B_N02_POL_I.Data1", "Dnet_B_N02_POL_I.Data2", "Dnet_B_N02_POL_I.ExtendedData", "Dnet_B_N02_POL_I.ExtendedData1", "Dnet_B_N02_POL_I.ExtendedData2", "Dnet_B_N02_POL_I.ExtendedData3", "Dnet_B_N02_POL_I.ExtendedData4", "Dnet_B_N03_POL_I.Data", "Dnet_B_N03_POL_I.Data1", "Dnet_B_N03_POL_I.Data2", "Dnet_B_N03_POL_I.ExtendedData", "Dnet_B_N03_POL_I.ExtendedData1", "Dnet_B_N03_POL_I.ExtendedData2", "Dnet_B_N03_POL_I.ExtendedData3", "Dnet_B_N03_POL_I.ExtendedData4", "Dnet_B_N04_POL_I.Data", "Dnet_B_N04_POL_I.Data1", "Dnet_B_N04_POL_I.Data2", "Dnet_B_N04_POL_I.ExtendedData", "Dnet_B_N04_POL_I.ExtendedData1", "Dnet_B_N04_POL_I.ExtendedData2", "Dnet_B_N04_POL_I.ExtendedData3", "Dnet_B_N04_POL_I.ExtendedData4", "Dnet_B_N05_POL_I.Data", "Dnet_B_N05_POL_I.Data1", "Dnet_B_N05_POL_I.Data2", "Dnet_B_N05_POL_I.ExtendedData", "Dnet_B_N05_POL_I.ExtendedData1", "Dnet_B_N05_POL_I.ExtendedData2", "Dnet_B_N05_POL_I.ExtendedData3", "Dnet_B_N05_POL_I.ExtendedData4", "Dnet_B_N06_POL_I.Data", "Dnet_B_N06_POL_I.Data1", "Dnet_B_N06_POL_I.Data2", "Dnet_B_N06_POL_I.ExtendedData", "Dnet_B_N06_POL_I.ExtendedData1", "Dnet_B_N06_POL_I.ExtendedData2", "Dnet_B_N06_POL_I.ExtendedData3", "Dnet_B_N06_POL_I.ExtendedData4", "Dnet_B_N08_POL_I.Data", "Dnet_B_N08_POL_I.Data1", "Dnet_B_N08_POL_I.Data2", "Dnet_B_N08_POL_I.ExtendedData", "Dnet_B_N08_POL_I.ExtendedData1", "Dnet_B_N08_POL_I.ExtendedData2", "Dnet_B_N08_POL_I.ExtendedData3", "Dnet_B_N08_POL_I.ExtendedData4", "Dnet_B_N09_POL_I.Data", "Dnet_B_N09_POL_I.Data1", "Dnet_B_N09_POL_I.Data2", "Dnet_B_N09_POL_I.ExtendedData", "Dnet_B_N09_POL_I.ExtendedData1", "Dnet_B_N09_POL_I.ExtendedData2", "Dnet_B_N09_POL_I.ExtendedData3", "Dnet_B_N09_POL_I.ExtendedData4", "Dnet_B_N10_POL_I.Data", "Dnet_B_N10_POL_I.Data1", "Dnet_B_N10_POL_I.Data2", "Dnet_B_N10_POL_I.ExtendedData", "Dnet_B_N10_POL_I.ExtendedData1", "Dnet_B_N10_POL_I.ExtendedData2", "Dnet_B_N10_POL_I.ExtendedData3", "Dnet_B_N10_POL_I.ExtendedData4", "Dnet_B_N11_POL_I.Data", "Dnet_B_N11_POL_I.Data1", "Dnet_B_N11_POL_I.Data2", "Dnet_B_N11_POL_I.ExtendedData", "Dnet_B_N11_POL_I.ExtendedData1", "Dnet_B_N11_POL_I.ExtendedData2", "Dnet_B_N11_POL_I.ExtendedData3", "Dnet_B_N11_POL_I.ExtendedData4", "Dnet_B_N12_POL_I.Data", "Dnet_B_N12_POL_I.Data1", "Dnet_B_N12_POL_I.Data2", "Dnet_B_N12_POL_I.ExtendedData", "Dnet_B_N12_POL_I.ExtendedData1", "Dnet_B_N12_POL_I.ExtendedData2", "Dnet_B_N12_POL_I.ExtendedData3", "Dnet_B_N12_POL_I.ExtendedData4", "Dnet_B_N13_POL_I.Data", "Dnet_B_N13_POL_I.Data1", "Dnet_B_N13_POL_I.Data2", "Dnet_B_N13_POL_I.ExtendedData", "Dnet_B_N13_POL_I.ExtendedData1", "Dnet_B_N13_POL_I.ExtendedData2", "Dnet_B_N13_POL_I.ExtendedData3", "Dnet_B_N13_POL_I.ExtendedData4", "Dnet_B_N14_POL_I.Data", "Dnet_B_N14_POL_I.Data1", "Dnet_B_N14_POL_I.Data2", "Dnet_B_N14_POL_I.ExtendedData", "Dnet_B_N14_POL_I.ExtendedData1", "Dnet_B_N14_POL_I.ExtendedData2", "Dnet_B_N14_POL_I.ExtendedData3", "Dnet_B_N14_POL_I.ExtendedData4", "Dnet_B_N15_POL_I.Data", "Dnet_B_N15_POL_I.Data1", "Dnet_B_N15_POL_I.Data2", "Dnet_B_N15_POL_I.ExtendedData", "Dnet_B_N15_POL_I.ExtendedData1", "Dnet_B_N15_POL_I.ExtendedData2", "Dnet_B_N15_POL_I.ExtendedData3", "Dnet_B_N15_POL_I.ExtendedData4", "Dnet_B_N16_POL_I.Data_x.Data_0", "Dnet_B_N16_POL_I.Data_x.Data_1", "Dnet_B_N16_POL_I.Data_x.Data_2", "Dnet_B_N17_POL_I.Data_x.Data_0", "Dnet_B_N17_POL_I.Data_x.Data_1", "Dnet_B_N17_POL_I.Data_x.Data_2", "Dnet_B_N20_POL_I.Data_x.Data_0", "Dnet_B_N20_POL_I.Data_x.Data_1", "Dnet_B_N20_POL_I.Data_x.Data_2", "Dnet_B_N21_POL_I.Data_x.Data_0", "Dnet_B_N21_POL_I.Data_x.Data_1", "Dnet_B_N21_POL_I.Data_x.Data_2", "Dnet_B_N22_POL_I.Data_x.Data_0", "Dnet_B_N22_POL_I.Data_x.Data_1", "Dnet_B_N22_POL_I.Data_x.Data_2", "Dnet_B_N22_POL_I.Data_x.Data_3", "Dnet_B_N22_POL_I.Data_x.Data_4", "Dnet_C_N09_POL_I.Data_x.Data_00", "Dnet_C_N09_POL_I.Data_x.Data_01", "Dnet_C_N09_POL_I.Data_x.Data_02", "Dnet_C_N09_POL_I.Data_x.Data_03", "Dnet_C_N09_POL_I.Data_x.Data_04", "Dnet_C_N09_POL_I.Data_x.Data_05", "Dnet_C_N09_POL_I.Data_x.Data_06", "Dnet_C_N09_POL_I.Data_x.Data_07", "Dnet_C_N09_POL_I.Data_x.Data_08", "Dnet_C_N09_POL_I.Data_x.Data_09", "Dnet_C_N09_POL_I.Data_x.Data_10", "Dnet_C_N09_POL_I.Data_x.Data_11", "Dnet_C_N09_POL_I.Data_x.Data_12", "Dnet_C_N09_POL_I.Data_x.Data_13", "Dnet_C_N09_POL_I.Data_x.Data_14", "Dnet_C_N09_POL_I.Data_x.Data_15", "Dnet_C_N09_POL_I.Data_x.Data_16", "Dnet_C_N09_POL_I.Data_x.Data_17", "Dnet_C_N09_POL_I.Data_x.Data_18", "Dnet_C_N09_POL_I.Data_x.Data_19", "Dnet_C_N09_POL_I.Data_x.Data_20", "Dnet_C_N09_POL_I.Data_x.Data_21", "Dnet_C_N09_POL_I.Data_x.Data_22", "Dnet_C_N09_POL_I.Data_x.Data_23", "Dnet_C_N09_POL_I.Data_x.Data_24", "Dnet_C_N09_POL_I.Data_x.Data_25", "Dnet_C_N09_POL_I.Data_x.Data_26", "Dnet_C_N09_POL_I.Data_x.Data_27", "Dnet_C_N09_POL_I.Data_x.Data_28", "Dnet_C_N09_POL_I.Data_x.Data_29", "Dnet_C_N09_POL_I.Data_x.Data_30", "Dnet_C_N09_POL_I.Data_x.Data_31", "Dnet_C_N09_POL_I.Data_x.Data_32", "Dnet_C_N09_POL_I.Data_x.Data_33", "Dnet_C_N09_POL_I.Data_x.Data_34", "Dnet_C_N09_POL_I.Data_x.Data_35", "Dnet_C_N09_POL_I.Data_x.Data_36", "Dnet_C_N09_POL_I.Data_x.Data_37", "Dnet_C_N09_POL_I.Data_x.Data_38", "Dnet_C_N09_POL_I.Data_x.Data_39", "Dnet_C_N09_POL_I.Data_x.Data_40", "Dnet_C_N09_POL_I.Data_x.Data_41", "Dnet_C_N09_POL_I.Data_x.Data_42", "Dnet_C_N09_POL_I.Data_x.Data_43", "Dnet_C_N09_POL_I.Data_x.Data_44", "Dnet_C_N09_POL_I.Data_x.Data_45", "Dnet_C_N09_POL_I.Data_x.Data_46", "Dnet_C_N09_POL_I.Data_x.Data_47", "Dnet_C_N09_POL_I.Data_x.Data_48", "Dnet_C_N09_POL_I.Data_x.Data_49", "Dnet_C_N09_POL_I.Data_x.Data_50", "Dnet_C_N09_POL_I.Data_x.Data_51", "Dnet_C_N09_POL_I.Data_x.Data_52", "Dnet_C_N09_POL_I.Data_x.Data_53", "Dnet_C_N09_POL_I.Data_x.Data_54", "Dnet_C_N09_POL_I.Data_x.Data_55", "Dnet_C_N09_POL_I.Data_x.Data_56", "Dnet_C_N09_POL_I.Data_x.Data_57", "Dnet_C_N09_POL_I.Data_x.Data_58", "Dnet_C_N09_POL_I.Data_x.Data_59", "Dnet_C_N09_POL_I.Data_x.Data_60", "Dnet_C_N09_POL_I.Data_x.Data_61", "Dnet_C_N09_POL_I.Data_x.Data_62", "Dnet_C_N09_POL_I.Data_x.Data_63", "Dnet_C_N09_POL_I.Data_x.Data_64", "Dnet_C_N09_POL_I.Data_x.Data_65", "Dnet_C_N09_POL_I.Data_x.Data_66", "Dnet_C_N09_POL_I.Data_x.Data_67", "Dnet_C_N09_POL_I.Data_x.Data_68", "Dnet_C_N09_POL_I.Data_x.Data_69", "Dnet_C_N09_POL_I.Data_x.Data_70", "Dnet_C_N09_POL_I.Data_x.Data_71", "Dnet_C_N09_POL_I.Data_x.Data_72", "Dnet_C_N09_POL_I.Data_x.Data_73", "Dnet_C_N09_POL_I.Data_x.Data_74", "Dnet_C_N09_POL_I.Data_x.Data_75", "Dnet_C_N09_POL_I.Data_x.Data_76", "Dnet_C_N09_POL_I.Data_x.Data_77", "Dnet_C_N09_POL_I.Data_x.Data_78", "Dnet_C_N09_POL_I.Data_x.Data_79", "Dnet_C_N09_POL_I.Data_x.Data_80", "Dnet_C_N09_POL_I.Data_x.Data_81", "Dnet_C_N09_POL_I.Data_x.Data_82", "Dnet_C_N09_POL_I.Data_x.Data_83"]  # DNet IO Input Strings
      w48 = string[][] [["Dnet", "Node", "Type", "ID Number", "SCCM", "FullScale", "Input Bytes", "Output Bytes"], ["A", "1", "MFC", "1", "200", "24576", "8", "2"], ["A", "2", "MFC", "44", "2000", "24576", "8", "2"], ["A", "3", "MFC", "45", "200", "24576", "8", "2"], ["A", "4", "PC", "10", "2000", "24576", "8", "2"], ["A", "5", "MFC", "2", "200", "24576", "8", "2"], ["A", "6", "MFC", "46", "2000", "24576", "8", "2"], ["A", "7", "MFC", "47", "200", "24576", "8", "2"], ["A", "8", "PC", "11", "2000", "24576", "8", "2"], ["A", "9", "MFC", "3", "1000", "24576", "8", "2"], ["A", "10", "PC", "12", "1000", "24576", "8", "2"], ["A", "11", "UNITMFC", "4", "500", "24576", "8", "2"], ["A", "12", "PC", "13", "500", "24576", "8", "2"], ["A", "13", "MFC", "5", "100", "24576", "8", "2"], ["A", "14", "MFC", "48", "1000", "24576", "8", "2"], ["A", "15", "MFC", "49", "100", "24576", "8", "2"], ["A", "16", "PC", "14", "1000", "24576", "8", "2"], ["A", "17", "MFC", "6", "100", "24576", "8", "2"], ["A", "19", "MFC", "51", "100", "24576", "8", "2"], ["A", "20", "PC", "15", "1000", "24576", "8", "2"], ["A", "21", "MFC", "7", "100", "24576", "8", "2"], ["A", "23", "MFC", "53", "100", "24576", "8", "2"], ["A", "24", "PC", "16", "1000", "24576", "8", "2"], ["A", "25", "MFC", "8", "200", "24576", "8", "2"], ["A", "27", "MFC", "55", "200", "24576", "8", "2"], ["A", "28", "PC", "17", "1000", "24576", "8", "2"], ["A", "29", "MFC", "9", "2000", "24576", "8", "2"], ["A", "31", "MFC", "37", "100", "24576", "8", "2"], ["A", "32", "MFC", "56", "500", "24576", "8", "2"], ["A", "33", "MFC", "33", "1000", "24576", "8", "2"], ["A", "34", "MFC", "32", "100", "24576", "8", "2"], ["A", "35", "MFC", "19", "9999999", "24576", "8", "2"], ["A", "36", "MFC", "20", "100", "24576", "8", "2"], ["A", "37", "UNITMFC", "52", "1000", "24576", "8", "2"], ["A", "38", "PC", "21", "9999999", "24576", "8", "2"], ["A", "39", "MFC", "22", "2000", "24576", "8", "2"], ["A", "40", "MFC", "23", "9999999", "24576", "8", "2"], ["A", "41", "PC", "24", "9999999", "24576", "8", "2"], ["A", "42", "MFC", "34", "9999999", "24576", "8", "2"], ["A", "43", "MFC", "35", "9999999", "24576", "8", "2"], ["A", "44", "MFC", "36", "100", "24576", "8", "2"], ["A", "45", "MFC", "38", "9999999", "24576", "8", "2"], ["A", "46", "MFC", "39", "9999999", "24576", "8", "2"], ["A", "47", "PC", "42", "2000", "24576", "8", "2"], ["A", "48", "BAR", "90", "0", "0", "3", "0"], ["A", "49", "RTPC", "29", "5000", "24576", "8", "3"], ["A", "50", "UNITMFC", "50", "1000", "24576", "8", "2"], ["A", "51", "UNITMFC", "54", "2000", "24576", "8", "2"], ["A", "52", "RTPC", "30", "9999999", "24576", "8", "3"], ["A", "53", "RTPC", "27", "5000", "24576", "8", "3"], ["A", "54", "RTPC", "28", "5000", "24576", "8", "3"], ["A", "55", "MFC", "57", "1000", "24576", "8", "2"], ["A", "56", "MFC", "41", "10", "24576", "8", "2"], ["A", "60", "TurboMotor", "0", "0", "0", "8", "8"], ["A", "61", "BAR", "91", "0", "0", "3", "0"], ["A", "63", "PC", "43", "500", "24576", "8", "2"], ["B", "1", "MFC", "78", "2000", "24576", "8", "2"], ["B", "2", "MFC", "79", "2000", "24576", "8", "2"], ["B", "3", "MFC", "80", "2000", "24576", "8", "2"], ["B", "4", "MFC", "83", "20000", "24576", "8", "2"], ["B", "5", "MFC", "81", "20000", "24576", "8", "2"], ["B", "6", "MFC", "82", "20000", "24576", "8", "2"], ["B", "8", "MFC", "68", "2000", "24576", "8", "2"], ["B", "9", "MFC", "85", "1000", "24576", "8", "2"], ["B", "10", "MFC", "69", "2000", "24576", "8", "2"], ["B", "11", "MFC", "86", "2000", "24576", "8", "2"], ["B", "12", "MFC", "70", "500", "24576", "8", "2"], ["B", "13", "MFC", "73", "1000", "24576", "8", "2"], ["B", "14", "MFC", "74", "1000", "24576", "8", "2"], ["B", "15", "MFC", "75", "5000", "24576", "8", "2"], ["B", "16", "BAR", "92", "0", "24576", "3", "0"], ["B", "17", "BAR", "93", "0", "24576", "3", "0"], ["B", "20", "BAR", "94", "0", "24576", "3", "0"], ["B", "21", "GP354", "0", "0", "0", "3", "1"], ["B", "22", "GP275", "0", "0", "0", "5", "0"], ["C", "9", "EZ-ZONE", "0", "0", "0", "84", "80"]]  # Dnet Map Strings
      w50 = string[] ["Local_2_O.CommandRegister.Run", "Local_2_O.CommandRegister.Fault", "Local_2_O.CommandRegister.DisableNetwork", "Local_2_O.CommandRegister.HaltScanner", "Local_2_O.CommandRegister.Reset", "Local_3_O.CommandRegister.Run", "Local_3_O.CommandRegister.Fault", "Local_3_O.CommandRegister.DisableNetwork", "Local_3_O.CommandRegister.HaltScanner", "Local_3_O.CommandRegister.Reset", "Local_4_O.CommandRegister.Run", "Local_4_O.CommandRegister.Fault", "Local_4_O.CommandRegister.DisableNetwork", "Local_4_O.CommandRegister.HaltScanner", "Local_4_O.CommandRegister.Reset"]  # DNet CommandRegister Strings
      w51 = string[] ["Local_2_S.DeviceFailureRegister_x.DeviceFailureRegister_0", "Local_2_S.DeviceFailureRegister_x.DeviceFailureRegister_1", "Local_2_S.DeviceFailureRegister_x.DeviceFailureRegister_2", "Local_2_S.DeviceFailureRegister_x.DeviceFailureRegister_3", "Local_2_S.DeviceFailureRegister_x.DeviceFailureRegister_4", "Local_2_S.DeviceFailureRegister_x.DeviceFailureRegister_5", "Local_2_S.DeviceFailureRegister_x.DeviceFailureRegister_6", "Local_2_S.DeviceFailureRegister_x.DeviceFailureRegister_7", "Local_2_S.AutoverifyFailureRegister_x.AutoverifyFailureRegister_0", "Local_2_S.AutoverifyFailureRegister_x.AutoverifyFailureRegister_1", "Local_2_S.AutoverifyFailureRegister_x.AutoverifyFailureRegister_2", "Local_2_S.AutoverifyFailureRegister_x.AutoverifyFailureRegister_3", "Local_2_S.AutoverifyFailureRegister_x.AutoverifyFailureRegister_4", "Local_2_S.AutoverifyFailureRegister_x.AutoverifyFailureRegister_5", "Local_2_S.AutoverifyFailureRegister_x.AutoverifyFailureRegister_6", "Local_2_S.AutoverifyFailureRegister_x.AutoverifyFailureRegister_7", "Local_2_S.DeviceIdleRegister_x.DeviceIdleRegister_0", "Local_2_S.DeviceIdleRegister_x.DeviceIdleRegister_1", "Local_2_S.DeviceIdleRegister_x.DeviceIdleRegister_2", "Local_2_S.DeviceIdleRegister_x.DeviceIdleRegister_3", "Local_2_S.DeviceIdleRegister_x.DeviceIdleRegister_4", "Local_2_S.DeviceIdleRegister_x.DeviceIdleRegister_5", "Local_2_S.DeviceIdleRegister_x.DeviceIdleRegister_6", "Local_2_S.DeviceIdleRegister_x.DeviceIdleRegister_7", "Local_2_S.ActiveNodeRegister_x.ActiveNodeRegister_0", "Local_2_S.ActiveNodeRegister_x.ActiveNodeRegister_1", "Local_2_S.ActiveNodeRegister_x.ActiveNodeRegister_2", "Local_2_S.ActiveNodeRegister_x.ActiveNodeRegister_3", "Local_2_S.ActiveNodeRegister_x.ActiveNodeRegister_4", "Local_2_S.ActiveNodeRegister_x.ActiveNodeRegister_5", "Local_2_S.ActiveNodeRegister_x.ActiveNodeRegister_6", "Local_2_S.ActiveNodeRegister_x.ActiveNodeRegister_7", "Local_2_S.StatusDisplay_x.StatusDisplay_0", "Local_2_S.StatusDisplay_x.StatusDisplay_1", "Local_2_S.StatusDisplay_x.StatusDisplay_2", "Local_2_S.StatusDisplay_x.StatusDisplay_3", "Local_2_S.ScannerAddress", "Local_2_S.ScannerStatus", "Local_2_S.ScrollingDeviceAddress", "Local_2_S.ScrollingDeviceStatus", "Local_3_S.DeviceFailureRegister_x.DeviceFailureRegister_0", "Local_3_S.DeviceFailureRegister_x.DeviceFailureRegister_1", "Local_3_S.DeviceFailureRegister_x.DeviceFailureRegister_2", "Local_3_S.DeviceFailureRegister_x.DeviceFailureRegister_3", "Local_3_S.DeviceFailureRegister_x.DeviceFailureRegister_4", "Local_3_S.DeviceFailureRegister_x.DeviceFailureRegister_5", "Local_3_S.DeviceFailureRegister_x.DeviceFailureRegister_6", "Local_3_S.DeviceFailureRegister_x.DeviceFailureRegister_7", "Local_3_S.AutoverifyFailureRegister_x.AutoverifyFailureRegister_0", "Local_3_S.AutoverifyFailureRegister_x.AutoverifyFailureRegister_1", "Local_3_S.AutoverifyFailureRegister_x.AutoverifyFailureRegister_2", "Local_3_S.AutoverifyFailureRegister_x.AutoverifyFailureRegister_3", "Local_3_S.AutoverifyFailureRegister_x.AutoverifyFailureRegister_4", "Local_3_S.AutoverifyFailureRegister_x.AutoverifyFailureRegister_5", "Local_3_S.AutoverifyFailureRegister_x.AutoverifyFailureRegister_6", "Local_3_S.AutoverifyFailureRegister_x.AutoverifyFailureRegister_7", "Local_3_S.DeviceIdleRegister_x.DeviceIdleRegister_0", "Local_3_S.DeviceIdleRegister_x.DeviceIdleRegister_1", "Local_3_S.DeviceIdleRegister_x.DeviceIdleRegister_2", "Local_3_S.DeviceIdleRegister_x.DeviceIdleRegister_3", "Local_3_S.DeviceIdleRegister_x.DeviceIdleRegister_4", "Local_3_S.DeviceIdleRegister_x.DeviceIdleRegister_5", "Local_3_S.DeviceIdleRegister_x.DeviceIdleRegister_6", "Local_3_S.DeviceIdleRegister_x.DeviceIdleRegister_7", "Local_3_S.ActiveNodeRegister_x.ActiveNodeRegister_0", "Local_3_S.ActiveNodeRegister_x.ActiveNodeRegister_1", "Local_3_S.ActiveNodeRegister_x.ActiveNodeRegister_2", "Local_3_S.ActiveNodeRegister_x.ActiveNodeRegister_3", "Local_3_S.ActiveNodeRegister_x.ActiveNodeRegister_4", "Local_3_S.ActiveNodeRegister_x.ActiveNodeRegister_5", "Local_3_S.ActiveNodeRegister_x.ActiveNodeRegister_6", "Local_3_S.ActiveNodeRegister_x.ActiveNodeRegister_7", "Local_3_S.StatusDisplay_x.StatusDisplay_0", "Local_3_S.StatusDisplay_x.StatusDisplay_1", "Local_3_S.StatusDisplay_x.StatusDisplay_2", "Local_3_S.StatusDisplay_x.StatusDisplay_3", "Local_3_S.ScannerAddress", "Local_3_S.ScannerStatus", "Local_3_S.ScrollingDeviceAddress", "Local_3_S.ScrollingDeviceStatus", "Local_4_S.DeviceFailureRegister_x.DeviceFailureRegister_0", "Local_4_S.DeviceFailureRegister_x.DeviceFailureRegister_1", "Local_4_S.DeviceFailureRegister_x.DeviceFailureRegister_2", "Local_4_S.DeviceFailureRegister_x.DeviceFailureRegister_3", "Local_4_S.DeviceFailureRegister_x.DeviceFailureRegister_4", "Local_4_S.DeviceFailureRegister_x.DeviceFailureRegister_5", "Local_4_S.DeviceFailureRegister_x.DeviceFailureRegister_6", "Local_4_S.DeviceFailureRegister_x.DeviceFailureRegister_7", "Local_4_S.AutoverifyFailureRegister_x.AutoverifyFailureRegister_0", "Local_4_S.AutoverifyFailureRegister_x.AutoverifyFailureRegister_1", "Local_4_S.AutoverifyFailureRegister_x.AutoverifyFailureRegister_2", "Local_4_S.AutoverifyFailureRegister_x.AutoverifyFailureRegister_3", "Local_4_S.AutoverifyFailureRegister_x.AutoverifyFailureRegister_4", "Local_4_S.AutoverifyFailureRegister_x.AutoverifyFailureRegister_5", "Local_4_S.AutoverifyFailureRegister_x.AutoverifyFailureRegister_6", "Local_4_S.AutoverifyFailureRegister_x.AutoverifyFailureRegister_7", "Local_4_S.DeviceIdleRegister_x.DeviceIdleRegister_0", "Local_4_S.DeviceIdleRegister_x.DeviceIdleRegister_1", "Local_4_S.DeviceIdleRegister_x.DeviceIdleRegister_2", "Local_4_S.DeviceIdleRegister_x.DeviceIdleRegister_3", "Local_4_S.DeviceIdleRegister_x.DeviceIdleRegister_4", "Local_4_S.DeviceIdleRegister_x.DeviceIdleRegister_5", "Local_4_S.DeviceIdleRegister_x.DeviceIdleRegister_6", "Local_4_S.DeviceIdleRegister_x.DeviceIdleRegister_7", "Local_4_S.ActiveNodeRegister_x.ActiveNodeRegister_0", "Local_4_S.ActiveNodeRegister_x.ActiveNodeRegister_1", "Local_4_S.ActiveNodeRegister_x.ActiveNodeRegister_2", "Local_4_S.ActiveNodeRegister_x.ActiveNodeRegister_3", "Local_4_S.ActiveNodeRegister_x.ActiveNodeRegister_4", "Local_4_S.ActiveNodeRegister_x.ActiveNodeRegister_5", "Local_4_S.ActiveNodeRegister_x.ActiveNodeRegister_6", "Local_4_S.ActiveNodeRegister_x.ActiveNodeRegister_7", "Local_4_S.StatusDisplay_x.StatusDisplay_0", "Local_4_S.StatusDisplay_x.StatusDisplay_1", "Local_4_S.StatusDisplay_x.StatusDisplay_2", "Local_4_S.StatusDisplay_x.StatusDisplay_3", "Local_4_S.ScannerAddress", "Local_4_S.ScannerStatus", "Local_4_S.ScrollingDeviceAddress", "Local_4_S.ScrollingDeviceStatus"]  # DNet Status Strings
      w52 = string[] ["Local_2_I.StatusRegister.Run", "Local_2_I.StatusRegister.Fault", "Local_2_I.StatusRegister.DisableNetwork", "Local_2_I.StatusRegister.DeviceFailure", "Local_2_I.StatusRegister.Autoverify", "Local_2_I.StatusRegister.CommFailure", "Local_2_I.StatusRegister.DupNodeFail", "Local_2_I.StatusRegister.DnetPowerDetect", "Local_3_I.StatusRegister.Run", "Local_3_I.StatusRegister.Fault", "Local_3_I.StatusRegister.DisableNetwork", "Local_3_I.StatusRegister.DeviceFailure", "Local_3_I.StatusRegister.Autoverify", "Local_3_I.StatusRegister.CommFailure", "Local_3_I.StatusRegister.DupNodeFail", "Local_3_I.StatusRegister.DnetPowerDetect", "Local_4_I.StatusRegister.Run", "Local_4_I.StatusRegister.Fault", "Local_4_I.StatusRegister.DisableNetwork", "Local_4_I.StatusRegister.DeviceFailure", "Local_4_I.StatusRegister.Autoverify", "Local_4_I.StatusRegister.CommFailure", "Local_4_I.StatusRegister.DupNodeFail", "Local_4_I.StatusRegister.DnetPowerDetect"]  # DNet StatusRegister Strings
      w53 = string[] ["Valve_x.Valve_000", "Valve_x.Valve_001", "Valve_x.Valve_002", "Valve_x.Valve_003", "Valve_x.Valve_004", "Valve_x.Valve_005", "Valve_x.Valve_006", "Valve_x.Valve_007", "Valve_x.Valve_008", "Valve_x.Valve_009", "Valve_x.Valve_010", "Valve_x.Valve_011", "Valve_x.Valve_012", "Valve_x.Valve_013", "Valve_x.Valve_014", "Valve_x.Valve_015", "Valve_x.Valve_016", "Valve_x.Valve_017", "Valve_x.Valve_018", "Valve_x.Valve_019", "Valve_x.Valve_020", "Valve_x.Valve_021", "Valve_x.Valve_022", "Valve_x.Valve_023", "Valve_x.Valve_024", "Valve_x.Valve_025", "Valve_x.Valve_026", "Valve_x.Valve_027", "Valve_x.Valve_028", "Valve_x.Valve_029", "Valve_x.Valve_030", "Valve_x.Valve_031", "Valve_x.Valve_032", "Valve_x.Valve_033", "Valve_x.Valve_034", "Valve_x.Valve_035", "Valve_x.Valve_036", "Valve_x.Valve_037", "Valve_x.Valve_038", "Valve_x.Valve_039", "Valve_x.Valve_040", "Valve_x.Valve_041", "Valve_x.Valve_042", "Valve_x.Valve_043", "Valve_x.Valve_044", "Valve_x.Valve_045", "Valve_x.Valve_046", "Valve_x.Valve_047", "Valve_x.Valve_048", "Valve_x.Valve_049", "Valve_x.Valve_050", "Valve_x.Valve_051", "Valve_x.Valve_052", "Valve_x.Valve_053", "Valve_x.Valve_054", "Valve_x.Valve_055", "Valve_x.Valve_056", "Valve_x.Valve_057", "Valve_x.Valve_058", "Valve_x.Valve_059", "Valve_x.Valve_060", "Valve_x.Valve_061", "Valve_x.Valve_062", "Valve_x.Valve_063", "Valve_x.Valve_064", "Valve_x.Valve_065", "Valve_x.Valve_066", "Valve_x.Valve_067", "Valve_x.Valve_068", "Valve_x.Valve_069", "Valve_x.Valve_070", "Valve_x.Valve_071", "Valve_x.Valve_072", "Valve_x.Valve_073", "Valve_x.Valve_074", "Valve_x.Valve_075", "Valve_x.Valve_076", "Valve_x.Valve_077", "Valve_x.Valve_078", "Valve_x.Valve_079", "Valve_x.Valve_080", "Valve_x.Valve_081", "Valve_x.Valve_082", "Valve_x.Valve_083", "Valve_x.Valve_084", "Valve_x.Valve_085", "Valve_x.Valve_086", "Valve_x.Valve_087", "Valve_x.Valve_088", "Valve_x.Valve_089", "Valve_x.Valve_090", "Valve_x.Valve_091", "Valve_x.Valve_092", "Valve_x.Valve_093", "Valve_x.Valve_094", "Valve_x.Valve_095", "Valve_x.Valve_096", "Valve_x.Valve_097", "Valve_x.Valve_098", "Valve_x.Valve_099", "Valve_x.Valve_100", "Valve_x.Valve_101", "Valve_x.Valve_102", "Valve_x.Valve_103", "Valve_x.Valve_104", "Valve_x.Valve_105", "Valve_x.Valve_106", "Valve_x.Valve_107", "Valve_x.Valve_108", "Valve_x.Valve_109", "Valve_x.Valve_110", "Valve_x.Valve_111", "Valve_x.Valve_112", "Valve_x.Valve_113", "Valve_x.Valve_114", "Valve_x.Valve_115", "Valve_x.Valve_116", "Valve_x.Valve_117", "Valve_x.Valve_118", "Valve_x.Valve_119", "Valve_x.Valve_120", "Valve_x.Valve_121", "Valve_x.Valve_122", "Valve_x.Valve_123", "Valve_x.Valve_124", "Valve_x.Valve_125", "Valve_x.Valve_126", "Valve_x.Valve_127"]  # Valve Strings 2
      w54 = string[] ["Local_10_O.Data"]  # Dout Strings
      w55 = string[] ["Local_8_I.Data", "Local_9_I.Data", "Local_10_I.Data"]  # Din Strings
      w57 = string[] ["Local_5_I.Ch0Data", "Local_5_I.Ch1Data", "Local_5_I.Ch2Data", "Local_5_I.Ch3Data", "Local_5_I.Ch4Data", "Local_5_I.Ch5Data", "Local_5_I.Ch6Data", "Local_5_I.Ch7Data", "Local_5_I.Ch8Data", "Local_5_I.Ch9Data", "Local_5_I.Ch10Data", "Local_5_I.Ch11Data", "Local_5_I.Ch12Data", "Local_5_I.Ch13Data", "Local_5_I.Ch14Data", "Local_5_I.Ch15Data"]  # Ain1 Strings
      w56 = string[] ["Local_6_I.Ch0Data", "Local_6_I.Ch1Data", "Local_6_I.Ch2Data", "Local_6_I.Ch3Data", "Local_6_I.Ch4Data", "Local_6_I.Ch5Data", "Local_6_I.Ch6Data", "Local_6_I.Ch7Data", "Local_6_I.Ch8Data", "Local_6_I.Ch9Data", "Local_6_I.Ch10Data", "Local_6_I.Ch11Data", "Local_6_I.Ch12Data", "Local_6_I.Ch13Data", "Local_6_I.Ch14Data", "Local_6_I.Ch15Data"]  # Ain2 Strings
      n32 = global write "GlobalVariables.vi" "DNet StatusRegister Strings"(w52) -> ()
      n33 = global write "GlobalVariables.vi" "DNet ScanCounter Strings"(string[] ["Local_2_S.ScanCounter", "Local_3_S.ScanCounter", "Local_4_S.ScanCounter"]) -> ()
      n34 = global write "GlobalVariables.vi" "DNet Status Strings"(w51) -> ()
      n35 = global write "GlobalVariables.vi" "DNet CommandRegister Strings"(w50) -> ()
      n36 = global write "GlobalVariables.vi" "Dnet Map Strings"(w48) -> ()
      n37 = global write "GlobalVariables.vi" "Dnet Input Strings"(w46) -> ()
      n38 = global write "GlobalVariables.vi" "Dnet Output Strings"(w47) -> ()
      n39 = global write "GlobalVariables.vi" "Ain1 Strings"(w57) -> ()
      n40 = global write "GlobalVariables.vi" "Ain2 Strings"(w56) -> ()
      n41 = global write "GlobalVariables.vi" "Din Strings"(w55) -> ()
      n42 = global write "GlobalVariables.vi" "Dout Strings"(w54) -> ()
      n43 = global write "GlobalVariables.vi" "Valve Strings 2"(w53) -> ()
    }
    frame #2 {
      w58 = 0 ("Output Bytes Counter")
      w63 = T6 {"Dnet"="", "Node"=0, "Type"="", "ID Number"=0, "SCCM"=0.0, "FullScale"=0.0, "Input Bytes"=0, "Output Bytes"=0, "Input Start Location"=0, "Output Start Location"=0, "Enabled"=TRUE, "Bytes"=[0, 0, 0]}  # Device Cluster
      n44 = global read "GlobalVariables.vi" "Dnet Map Strings"() -> (w60:string[][])
      n45 = for {
        tunnel: w63 -> [w85]
        tunnel: [w84] -> w59 mode=indexing
        tunnel: w60 -> [w74] mode=indexing
        shift-right: [w64] -> _
        shift-left: w58 -> [w67]
        shift-right: [w65] -> _
        shift-left: w58 -> [w66]
        w79 = 0.0
        n46 = Index Array(array=w74) -> (element #1=w78:string, element #2=w77:string, element #3=w76:string, element #4=w75:string, element #5=w73:string, element #6=w72:string, element #7=w71:string, element #8=w70:string)  [unwired: 8 in]
        n47 = Decimal String To Number(string=w75) -> (number=w82:i32)  [unwired: 2 in, 1 out]
        n48 = Decimal String To Number(string=w73, default (0L)=w79) -> (number=w81:dbl)  [unwired: 1 in, 1 out]
        n49 = Decimal String To Number(string=w72, default (0L)=w79) -> (number=w80:dbl)  [unwired: 1 in, 1 out]
        n50 = Decimal String To Number(string=w71) -> (number=w69:i32)  [unwired: 2 in, 1 out]
        n51 = Decimal String To Number(string=w70) -> (number=w68:i32)  [unwired: 2 in, 1 out]
        n52 = Decimal String To Number(string=w77) -> (number=w83:i32)  [unwired: 2 in, 1 out]
        n53 = Bundle By Name(cluster=w85, "Dnet"=w78, "Node"=w83, "Type"=w76, "ID Number"=w82, "SCCM"=w81, "FullScale"=w80, "Input Bytes"=w69, "Output Bytes"=w68, "Input Start Location"=w67, "Output Start Location"=w66) -> (w84:T6)
        n54 = Add(x=w67, y=w69) -> (x+y=w64:i32)
        n55 = Add(x=w66, y=w68) -> (x+y=w65:i32)
      }
      n56 = Delete From Array(array=w59, index=0) -> (array with subset deleted=w61:T6[])  [unwired: 1 in, 1 out]
      n57 = global write "GlobalVariables.vi" "Devices"(w61) -> ()
    }
    frame #3 {
      n58 = global read "GlobalVariables.vi" "Devices"() -> (w87:T6[])
      n59 = for {
        tunnel: w87 -> [w91] mode=indexing
        tunnel: [w92] -> w86 mode=indexing
        n60 = Unbundle By Name(w91) -> ("Bytes"=w89:u8[], "Output Bytes"=w88:i32)
        n61 = Reshape Array(w89, w88) -> (w90:u8[])
        n62 = Bundle By Name(cluster=w91, "Bytes"=w90) -> (w92:T6)
      }
      n63 = global write "GlobalVariables.vi" "Devices"(w86) -> ()
    }
  }
